vi "StripInt.vi"(2 "Width":i32=4, 3 "String":string) -> (0 "Remaining":string, 1 "Value":u32)   [LabVIEW 2011]
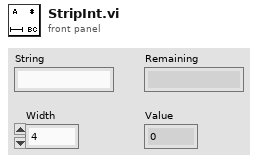
[diagram p1: front panel]
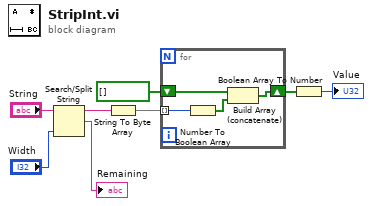
[diagram p0: block diagram]
diagram:
  n1 = Search/Split String(string="String", offset (0)="Width") -> (substring before match=w2:string, match + rest of string=→"Remaining":string)  [unwired: 1 in, 1 out]
  n2 = String To Byte Array(string=w2) -> (unsigned byte array=w5:u8[])
  n3 = for {
    tunnel: w5 -> [w12] mode=indexing
    shift-right: [w10] -> w6
    shift-left: bool[] [] ("Boolean array") -> [w9]
    n4 = Number To Boolean Array(number=w12) -> (Boolean array=w11:bool[])
    n5 = Build Array (concatenate)(w9, w11) -> (w10:bool[])
  }
  n6 = Boolean Array To Number(Boolean array=w6) -> (number=→"Value":u32)
